vi "Advanced Parallel Pressure Control.vi"() -> ()   [LabVIEW 2016]
doc: "Purpose: This example shows how to send concurrent pressure orders using threads. Dll handle parallel calls, functions can be called simultaneous. This demonstrate thread handling, same result is obtained using successive calls as al functions call is executed instantly (within few µs)\nHardware setup: At least two Fluigent pressure controllers (MFCS, MFCS-EZ or FlowEZ)"
uses:
  fgt_SDK.lvlib
panel:
  out "Stopped ?":bool
  out "Pressure chart":cluster{"element":sgl, "pressure out":sgl}(graph)
  in  "Stop":bool
  out "error out":errorcluster
  # "Hit the \"Run\" button to start generating pressure"
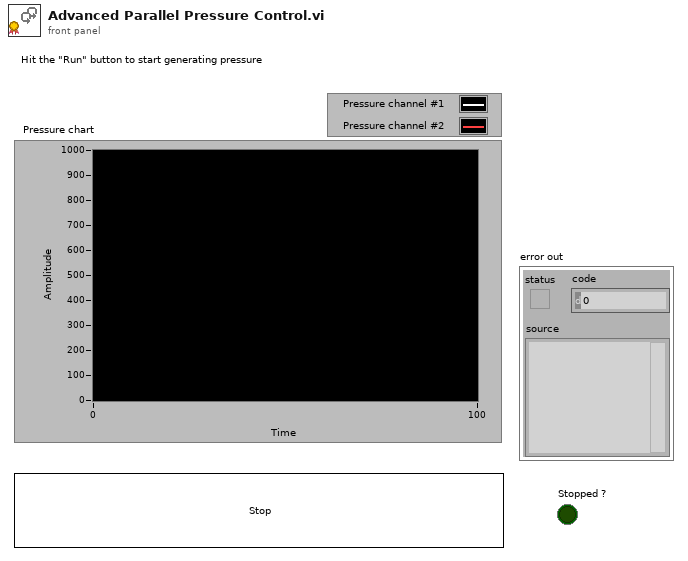
[diagram p1: front panel]
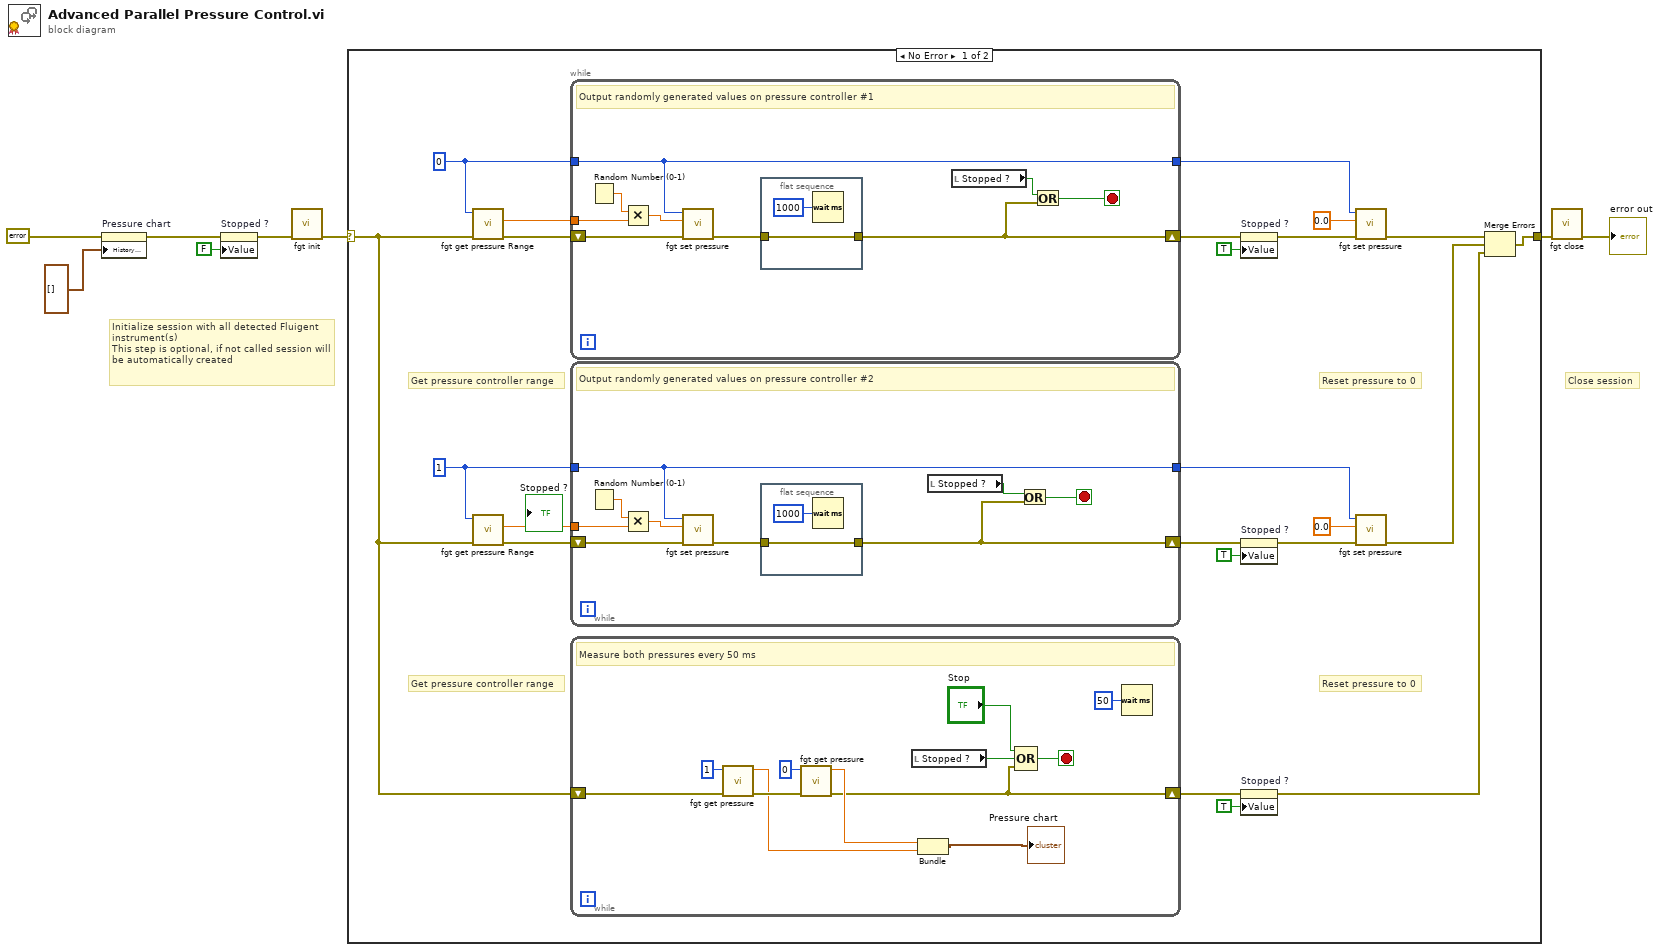
[diagram p0: block diagram]
diagram:
  # "Close session"
  # "Initialize session with all detected Fluigent instrument(s)\nThis step is optional, if not called session will be automatically created"
  n1 = property on="Pressure chart" class="WFChart (strict)"(error in=errorcluster {"status"=FALSE, "code"=0, "source"=""} ("error in (no error)"), "History Data"=cluster{"element":sgl, "pressure out":sgl}[] []) -> (error out=w3:errorcluster)  [unwired: 1 in, 1 out]
  n2 = property on="Stopped ?" class="Bool (strict)"(error in=w3, "Value"=FALSE ("Stop")) -> (error out=w5:errorcluster)  [unwired: 1 in, 1 out]
  n3 = call "fgt init.vi"("error in (no error)"=w5) -> ("error out"=w8:errorcluster)  [unwired: 10 in]
  n4 = case shown="No Error" w8 {
    selector: w8 -> [w18 w65]
    tunnel: [w20 w65] -> w7
    frame No Error {
      w24 = u32 1 ("pressureIndex")
      w27 = u32 0 ("pressureIndex")
      # "Reset pressure to 0"
      # "Get pressure controller range"
      # "Reset pressure to 0"
      # "Get pressure controller range"
      n5 = call "fgt get pressure Range.vi"("error in (no error)"=w18, "pressureIndex"=w27) -> ("error out"=w31:errorcluster, "Pmax out"=w28:sgl)  [unwired: 7 in, 1 out]
      n6 = call "fgt get pressure Range.vi"("error in (no error)"=w18, "pressureIndex"=w24) -> ("error out"=w21:errorcluster, "Pmax out"=w23:sgl)  [unwired: 7 in, 1 out]
      n7 = while {
        shift-right: [w56] -> w17
        shift-left: w31 -> [w62]
        tunnel: w28 -> [w59]
        tunnel: w27 -> [w57]
        tunnel: [w57] -> w26
        stop <- w55 stop-if-true
        # "Output randomly generated values on pressure controller #1"
        n8 = Random Number (0-1)() -> (number: 0 to 1=w60:dbl)
        n9 = Multiply(x=w60, y=w59) -> (x*y=w58:dbl)
        n10 = call "fgt set pressure.vi"("error in (no error)"=w62, "pressure"=w58, "pressureIndex"=w57) -> ("error out"=w61:errorcluster)  [unwired: 8 in]
        n11 = flat-sequence {
          tunnel: [w63] -> w56
          tunnel: w61 -> [w63]
          frame #0 {
            n12 = Wait (ms)(milliseconds to wait=u32 1000) -> ()  [unwired: 1 out]
          }
        }
        n13 = local read "Stopped ?"() -> (w54:bool)
        n14 = Or(x=w54, y=w56) -> (x .or. y?=w55:bool)
      }
      n15 = while {
        shift-right: [w45] -> w13
        shift-left: w21 -> [w51]
        tunnel: w23 -> [w48]
        tunnel: w24 -> [w46]
        tunnel: [w46] -> w25
        stop <- w44 stop-if-true
        # "Output randomly generated values on pressure controller #2"
        n16 = Random Number (0-1)() -> (number: 0 to 1=w49:dbl)
        n17 = Multiply(x=w49, y=w48) -> (x*y=w47:dbl)
        n18 = call "fgt set pressure.vi"("error in (no error)"=w51, "pressure"=w47, "pressureIndex"=w46) -> ("error out"=w50:errorcluster)  [unwired: 8 in]
        n19 = flat-sequence {
          tunnel: [w52] -> w45
          tunnel: w50 -> [w52]
          frame #0 {
            n20 = Wait (ms)(milliseconds to wait=u32 1000) -> ()  [unwired: 1 out]
          }
        }
        n21 = local read "Stopped ?"() -> (w43:bool)
        n22 = Or(x=w43, y=w45) -> (x .or. y?=w44:bool)
      }
      n23 = while {
        shift-right: [w33] -> w10
        shift-left: w18 -> [w42]
        stop <- w41 stop-if-true
        # "Measure both pressures every 50 ms"
        n24 = call "fgt get pressure.vi"("pressureIndex"=u32 1) -> ("pressure out"=w36:sgl)  [unwired: 9 in, 1 out]
        n25 = call "fgt get pressure.vi"("error in (no error)"=w42, "pressureIndex"=u32 0) -> ("error out"=w33:errorcluster, "pressure out"=w37:sgl)  [unwired: 8 in]
        n26 = local read "Stopped ?"() -> (w32:bool)
        n27 = Bundle("pressure out"=w37, "pressure out"=w36) -> (→"Pressure chart":cluster{"pressure out":sgl, "pressure out":sgl})  [unwired: 1 in]
        n28 = Compound Arithmetic op=OR("Stop", w32, w33) -> (w41:bool)
        n29 = Wait (ms)(milliseconds to wait=u32 50) -> ()  [unwired: 1 out]
      }
      n30 = property on="Stopped ?" class="Bool (strict)"(error in=w17, "Value"=TRUE ("Stop")) -> (error out=w16:errorcluster)  [unwired: 1 in, 1 out]
      n31 = property on="Stopped ?" class="Bool (strict)"(error in=w13, "Value"=TRUE ("Stop")) -> (error out=w12:errorcluster)  [unwired: 1 in, 1 out]
      n32 = property on="Stopped ?" class="Bool (strict)"(error in=w10, "Value"=TRUE ("Stop")) -> (error out=w9:errorcluster)  [unwired: 1 in, 1 out]
      n33 = call "fgt set pressure.vi"("error in (no error)"=w16, "pressure"=sgl 0.0, "pressureIndex"=w26) -> ("error out"=w29:errorcluster)  [unwired: 8 in]
      n34 = call "fgt set pressure.vi"("error in (no error)"=w12, "pressure"=sgl 0.0, "pressureIndex"=w25) -> ("error out"=w19:errorcluster)  [unwired: 8 in]
      n35 = Merge Errors(w29, w19, w9) -> (w20:errorcluster)
    }
    frame Error {
    }
  }
  n36 = call "fgt close.vi"("error in (no error)"=w7) -> ("error out"=→"error out":errorcluster)  [unwired: 10 in]
